vi "KIM_UI_launcher.vi"   [LabVIEW 2023]
uses:
  KIM101_Actor/KIM101_UI/KIM101_UI/KIM101_UI.lvclass
  <vilib>/ActorFramework/Actor/Actor.lvclass
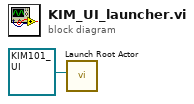
[diagram p0: block diagram]
diagram:
  n1 = call <vilib>:"Launch Root Actor.vi"("Actor"=refnum<class "KIM101_UI.lvclass"> refnum ("KIM101_UI.lvlib:KIM101_UI.lvclass")) -> ()  [unwired: 9 in, 2 out]
